vi "XY-READ.vi"(8 "Error IN":errorcluster, 10 "X/Y ?":enum16{"X", "Y"}(ring), 11 "SR850 GPIB IN":refnum<visa-resource-name>) -> (0 "Error OUT":errorcluster, 2 "SR850_Reading":dbl, 3 "SR850 GPIB OUT":refnum<visa-resource-name>)   [LabVIEW 2014]
panel:
  out "array":dbl[](array[numeric])
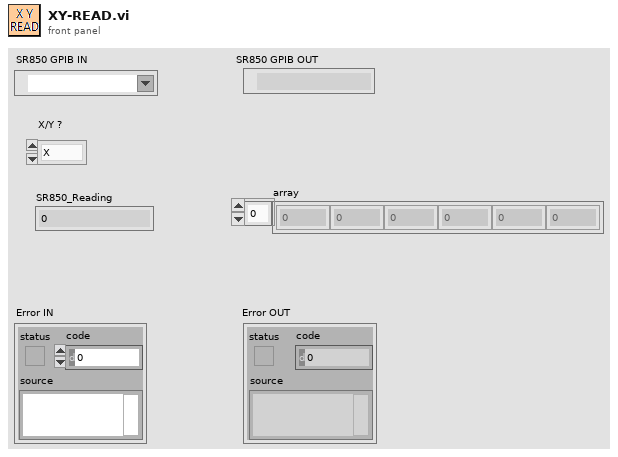
[diagram p1: front panel]
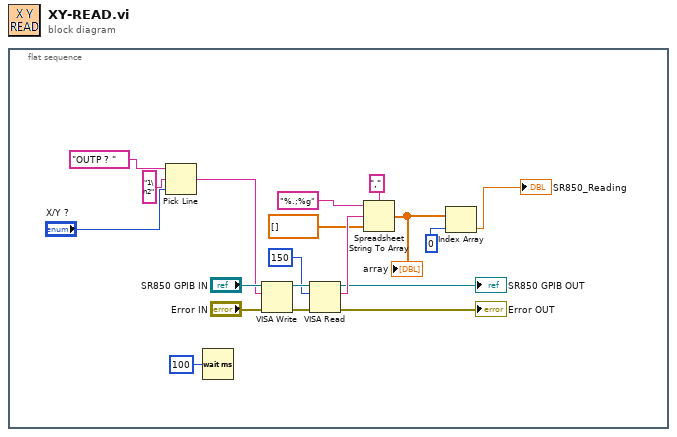
[diagram p0: block diagram]
diagram:
  n1 = flat-sequence {
    frame #0 {
      n2 = Pick Line(string ("")="OUTP ? " ("write buffer"), multi-line string="1\n2", line index="X/Y ?") -> (output string=w5:string)
      n3 = Wait (ms)(milliseconds to wait=u32 100) -> ()  [unwired: 1 out]
      n4 = VISA Write(VISA resource name="SR850 GPIB IN", write buffer=w5, error in (no error)="Error IN") -> (VISA resource name out=w16:refnum<visa-resource-name>, error out=w17:errorcluster)  [unwired: 1 out]
      n5 = VISA Read(VISA resource name=w16, byte count=u32 150, error in (no error)=w17) -> (VISA resource name out=→"SR850 GPIB OUT":refnum<visa-resource-name>, read buffer=w14:string, error out=→"Error OUT":errorcluster)  [unwired: 1 out]
      n6 = Spreadsheet String To Array(delimiter (Tab)=",", format string="%.;%g", spreadsheet string=w14, array type (2D Dbl)=dbl[] []) -> (array=w4:dbl[])
      "array" <- w4
      n7 = Index Array(array=w4, index=0) -> (element=→"SR850_Reading":dbl)
    }
  }
